vi "Tester_Task Setting Editor.vi"() -> ()   [LabVIEW 2017]
uses:
  Task Setting Editor/Task Setting Editor.lvclass/Task Setting Editor.ctl
  WebSocket Server/Actors/Actor wHelper/Actor wHelper/Actor wHelper.lvclass/Actor wHelper.ctl
  Task Setting Editor Messages/Set Task List Msg/Set Task List Msg.lvclass/Set Task List Msg.ctl
  <vilib>/ActorFramework/Message Enqueuer/Message Enqueuer.lvclass/Message Enqueuer.ctl
  Task Setting Editor Messages/Populate Worker Ring Msg/Populate Worker Ring Msg.lvclass/Populate Worker Ring Msg.ctl
  Task Setting Editor Messages/Open FrontPanel Msg/Open FrontPanel Msg.lvclass/Open FrontPanel Msg.ctl
  BuildWorker/Classes/Task/Task.lvclass/Task.ctl
  BuildWorker/Classes/Task/Get Name.vi
  BuildWorker/Classes/Task/Read Worker.vi
  Task Setting Editor/Read Task Updated.vi
  WebSocket Server/Actors/Actor wHelper/Actor wHelper/Read StopHelperLoop Reg Ref.vi
  <vilib>/ActorFramework/Message Enqueuer/Enqueue.vi
  Task Setting Editor/Task Setting Editor.lvclass
  Applications/National Instruments/LabVIEW 2017 64-bit/vi.lib/ActorFramework/Actor/Actor.lvclass
  Volumes/Data/Users/benji667/Git/BuildFarm/WebSocket Server/Actors/Actor wHelper/Actor wHelper/Actor wHelper.lvclass
  Task Setting Editor Messages/Set Task List Msg/Set Task List Msg.lvclass
  Applications/National Instruments/LabVIEW 2017 64-bit/vi.lib/ActorFramework/Message/Message.lvclass
  Task Setting Editor Messages/Populate Worker Ring Msg/Populate Worker Ring Msg.lvclass
  Task Setting Editor Messages/Open FrontPanel Msg/Open FrontPanel Msg.lvclass
  <vilib>/ActorFramework/Stop Msg/Stop Msg.lvclass
  <vilib>/ActorFramework/Message Priority Queue/Priority Enqueue.vi
  BuildWorker/Classes/Task/Task.lvclass
  <vilib>/ActorFramework/Actor/Actor.lvclass
  <vilib>/ActorFramework/Message Enqueuer/Message Enqueuer.lvclass
panel:
  out "Array 2":string[](array[string])
  out "Array":string[](array[string])
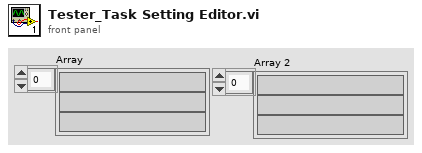
[diagram p1: front panel]
types:
  T1 = cluster{"Event Registration Refnum":refnum<event-registration>, "Properties:StopHelperLoop Reg Ref":refnum<event-registration>}
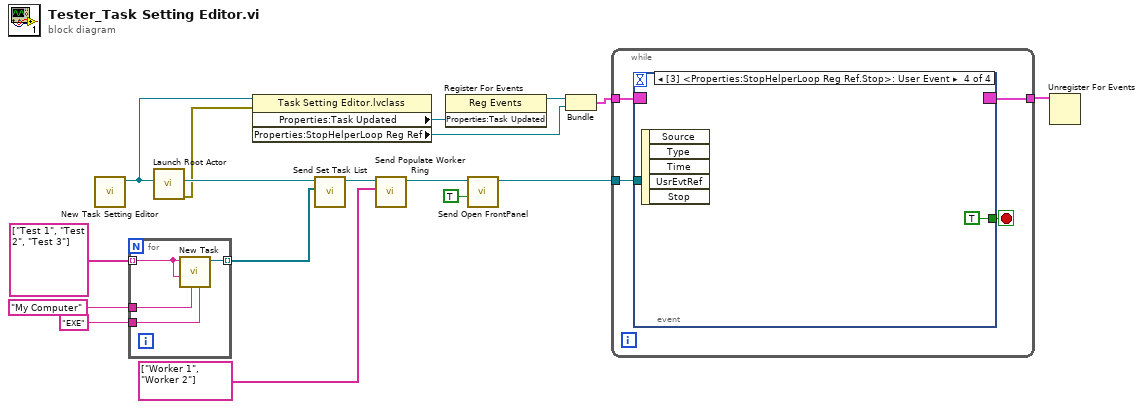
[diagram p0: block diagram]
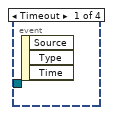
[diagram p2: hidden frame]
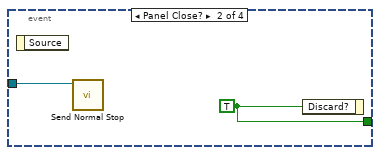
[diagram p3: hidden frame]
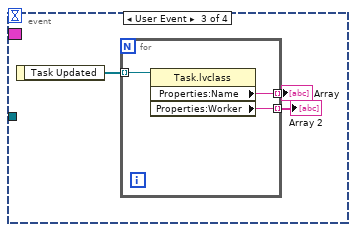
[diagram p4: hidden frame]
diagram:
  n1 = call "New Task Setting Editor.vi"() -> ("Task Setting Editor out"=w1:refnum<class "Task Setting Editor.lvclass">)  [unwired: 10 in, 1 out]
  n2 = for {
    tunnel: string[] ["Test 1", "Test 2", "Test 3"] -> [w21] mode=indexing
    tunnel: "My Computer" ("Target") -> [w20]
    tunnel: "EXE" ("Target") -> [w19]
    tunnel: [w18] -> w13 mode=indexing
    n3 = call "New Task.vi"("BuildSpec Type"=w19, "Target"=w20, "BuildSpec Name"=w21, "Name"=w21) -> ("Task out"=w18:refnum<class "Task.lvclass">)  [unwired: 6 in, 1 out]
  }
  n4 = call <vilib>:"Launch Root Actor.vi"("Actor"=w1) -> ("error out"=w2:errorcluster, "Actor's Enqueuer"=w14:refnum<class "Message Enqueuer.lvclass">)  [unwired: 9 in]
  n5 = property class="Task Setting Editor.lvclass"(reference=w1, error in=w2) -> ("Properties:Task Updated"=w5:refnum<user-event>, "Properties:StopHelperLoop Reg Ref"=w3:refnum<event-registration>)  [unwired: 2 out]
  n6 = call "Send Set Task List.vi"("Task List"=w13, "Message Enqueuer"=w14) -> ("Message Enqueuer out"=w12:refnum<class "Message Enqueuer.lvclass">)  [unwired: 8 in, 1 out]
  n7 = call "Send Populate Worker Ring.vi"("Worker List"=string[] ["Worker 1", "Worker 2"], "Message Enqueuer"=w12) -> ("Message Enqueuer out"=w8:refnum<class "Message Enqueuer.lvclass">)  [unwired: 8 in, 1 out]
  n8 = register-events(w5) -> (reference out=w10:refnum<event-registration>)  [unwired: 2 in, 1 out]
  n9 = call "Send Open FrontPanel.vi"("Open"=TRUE, "Message Enqueuer"=w8) -> ("Message Enqueuer out"=w7:refnum<class "Message Enqueuer.lvclass">)  [unwired: 8 in, 1 out]
  n10 = Bundle("Event Registration Refnum"=w10, "Properties:StopHelperLoop Reg Ref"=w3) -> (w4:T1)  [unwired: 1 in]
  n11 = while {
    tunnel: w4 -> [w25]
    tunnel: w7 -> [w24]
    tunnel: [w22] -> w9
    stop <- w23 stop-if-true
    n12 = event shown="[3] <Properties:StopHelperLoop Reg Ref.Stop>: User Event" {
      selector: w25 -> [_ _ _ _]
      dyn-events: [_ _ _ _] -> w22
      timeout: _ -> [_ _ _ _]
      tunnel: w24 -> [_ w26 _ _]
      tunnel: [_ w27 _ TRUE ("Discard?")] -> w23
      event Timeout {
        n13 = event-data() -> ()  [unwired: 1 in, 3 out]
      }
      event Panel Close? {
        w27 = TRUE ("Discard?")
        n14 = event-data() -> ()  [unwired: 1 in, 1 out]
        n15 = call <vilib>:"Send Normal Stop.vi"("Message Enqueuer"=w26) -> ()  [unwired: 10 in, 1 out]
        n16 = event-data("Discard?"=w27) -> ()  [unwired: 1 in, 1 out]
      }
      event User Event {
        n17 = event-data() -> ("Task Updated"=w30:refnum<class "Task.lvclass">[])  [unwired: 1 in]
        n18 = for {
          tunnel: w30 -> [w33] mode=indexing
          tunnel: [w32] -> w28 mode=indexing
          tunnel: [w31] -> w29 mode=indexing
          n19 = property class="Task.lvclass"(reference=w33) -> ("Properties:Name"=w31:string, "Properties:Worker"=w32:string)  [unwired: 1 in, 2 out]
        }
        "Array" <- w29
        "Array 2" <- w28
      }
      event User Event {
        n20 = event-data() -> ()  [unwired: 1 in, 5 out]
      }
    }
  }
  n21 = Unregister For Events(event registration refnum=w9) -> ()  [unwired: 1 in, 1 out]
